vi "StopRCM_RCM.vi"(0 "Display State In":T1={"RCM File Path"=path "", "Left"=300, "Top"=300, "Font Name"="Tahoma", "Font Size"=13, "Font Color"=0, "Separator Color"=9868950, "Frame Color"=9868950, "Overlay Color"=26367}, 9 "Container State":T2, 11 "error in (no error)":errorcluster) -> (4 "Display State Out":T1={"RCM File Path"=path "", "Left"=300, "Top"=300, "Font Name"="Tahoma", "Font Size"=13, "Font Color"=0, "Separator Color"=9868950, "Frame Color"=9868950, "Overlay Color"=26367}, 15 "error out":errorcluster)   [LabVIEW 2009, in "RCM.xctl"]
uses:
  RCM.xctl
  <vilib>/_xctls/Container State.ctl
  Ability/State_RCM.ctl
  <vilib>/_xctls/XControlSupport.lvlib
types:
  T1 = typedef "RCM.xctl/State_RCM.ctl" = cluster{"RCM File Path":path, "Left":u32, "Top":u32, "Font Name":string, "Font Size":i16, "Font Color":u32, "Separator Color":u32, "Frame Color":u32, "Overlay Color":u32}
  T2 = typedef "XControlSupport.lvlib/Container State.ctl" = cluster{"Indicator?":bool, "Run Mode?":bool, " Refnum":refnum<vi>}
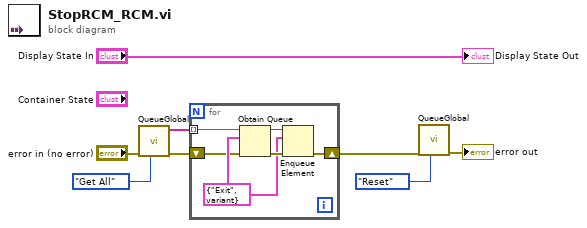
[diagram p0: block diagram]
diagram:
  n1 = call "QueueGlobal.vi"("cmd (Add)"=enum16{"Add One to End", "Get All", "Reset"}."Get All", "error in (no error)"="error in (no error)") -> ("error out"=w6:errorcluster, "queue names"=w3:string[])  [unwired: 8 in]
  n2 = for {
    shift-right: [w14] -> w5
    shift-left: w6 -> [w9]
    tunnel: w3 -> [w10] mode=indexing
    w11 = cluster{"State":string, "Data":variant} {"State"="Exit", "Data"=variant} ("element")
    n3 = Obtain Queue(name (unnamed)=w10, element data type=w11, error in (no error)=w9) -> (queue out=w13:refnum<queue>, error out=w12:errorcluster)  [unwired: 2 in, 1 out]
    n4 = Enqueue Element(queue=w13, element=w11, error in (no error)=w12) -> (error out=w14:errorcluster)  [unwired: 1 in, 2 out]
  }
  n5 = call "QueueGlobal.vi"("cmd (Add)"=enum16{"Add One to End", "Get All", "Reset"}."Reset", "error in (no error)"=w5) -> ("error out"=→"error out":errorcluster)  [unwired: 8 in, 1 out]
  "Display State Out" <- "Display State In"
